vi "SetDUTPosition.vi"(0 "reference in":refnum<class "MES_Local.lvclass">, 2 "DUTPosition":i32, 5 "error in (no error)":errorcluster) -> (14 "reference in":refnum<class "MES_Local.lvclass">, 19 "error out":errorcluster)   [LabVIEW 2022 SP3, in "MES_Local.lvlib" / "MES_Local.lvclass"]
uses:
  MES_Local.lvclass
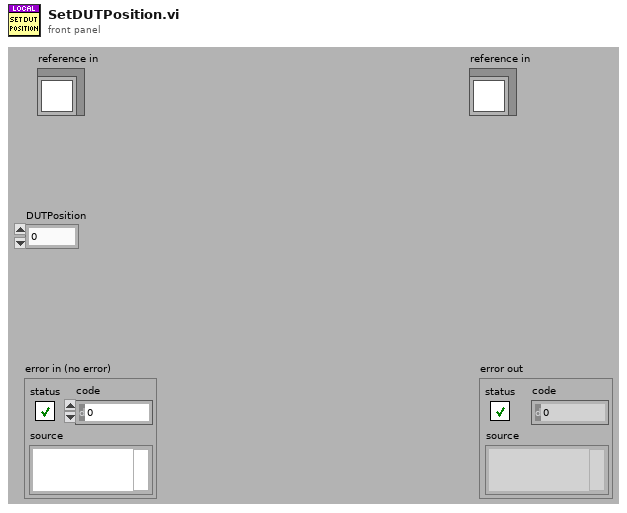
[diagram p1: front panel]
types:
  T1 = typedef "MES_Local.lvlib/MES_Local.lvclass/ObjectAttributes.ctl" = cluster{"Config":T2, "Logged_In?":bool, "AttributeNames":string[], "AttributeWritten":bool[], "ComponentNames":string[], "TestIndex":i32, "TestTag":string[], "Time Stamp":timestamp, "Employee":string, "Resource_Key":string, "Local Spec":path, "Login":refnum<class "Login_Base.lvclass">, "ReportPath":path, "Spec":T3, "StartTime":timestamp, "Role":string}
  T2 = typedef "MES_Local.lvlib/MES_Local.lvclass/Config.ctl" = cluster{"Results_Path":path}
  T3 = typedef "MES_Base.lvlibp/MES_Base.lvclass/Spec.ctl" = cluster{"Header":cluster{"Doctype":string, "Checksum":string, "DriverKey":string, "SpecId":string, "TransactionId":string, "AccountId":string, "SpecName":string, "WorkflowStep":string, "SerialNumber":string, "BatchNumber":string, "Status":enum16{"Pending", "Pass", "Fail"}, "Comment":string, "FirstFail":string, "Employee":string, "LocalMachine":string, "ResourceKey":string, "Date":string, "Time":string, "Duration":string, "DUT Position":i32}, "Components":cluster{"SerialNumber":string, "PartNumber":string, "Revision":string, "BatchNumber":string, "Name":string, "Description":string, "Attached":bool}[], "Attributes":cluster{"Name":string, "Description":string, "DataType":enum16{"NA", "String", "Boolean", "Int", "Dbl"}, "Value":variant, "DisplayFormat":string, "ReadOnly":bool, "Required":bool}[], "Tests":cluster{"Code":string, "Name":string, "Description":string, "Group":string, "IsGroup":bool, "Tag":string, "Method":string, "Parrameter":string, "DataType":enum16{"NA", "String", "Boolean", "Int", "Dbl"}, "Value":variant, "Status":enum16{"Pending", "Pass", "Fail"}, "LimitLo":variant, "LimitHi":variant, "StringMatch":string, "BooleanMatch":bool, "DisplayFormat":string, "Units":string, "TestTime":dbl}[]}
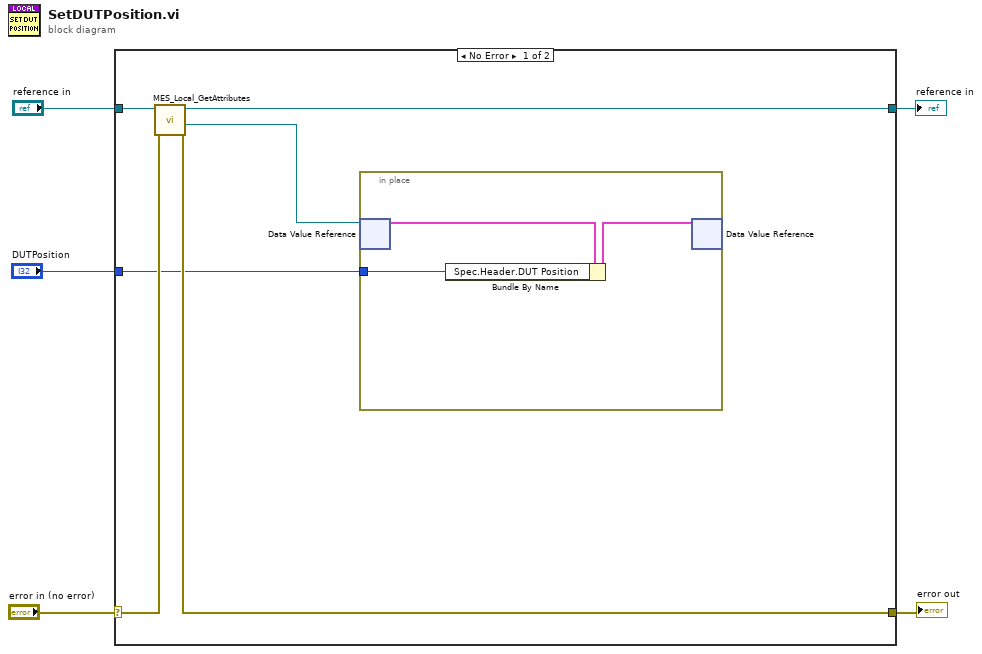
[diagram p0: block diagram]
diagram:
  n1 = case shown="No Error" "error in (no error)" {
    selector: "error in (no error)" -> [w11 w16]
    tunnel: [w10 w16] -> w4
    tunnel: [w8 w15] -> w2
    tunnel: "reference in" -> [w9 w15]
    tunnel: "DUTPosition" -> [w6 _]
    frame No Error {
      n2 = call "MES_Local_GetAttributes.vi"("error in (no error)"=w11, "reference in"=w9) -> ("error out"=w10:errorcluster, "DataRef"=w7:refnum<data-value>, "reference out"=w8:refnum<class "MES_Local.lvclass">)  [unwired: 6 in, 1 out]
      n3 = in-place {
        in-place-border: w6 -> [w12]
        n4 = in-place-dvr #1(w7) -> (w14:T1)  [unwired: 1 out]
        n5 = Bundle By Name(cluster=w14, "Spec.Header.DUT Position"=w12) -> (w13:T1)
        n6 = in-place-dvr #1(w13) -> ()  [unwired: 2 out]
      }
    }
    frame Error {
    }
  }
  "error out" <- w4
  "reference in" <- w2
